vi "Test4_udp.vi"() -> ()   [LabVIEW 2014]
panel:
  out "Numeric":dbl
  in  "stop":bool
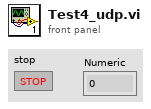
[diagram p1: front panel]
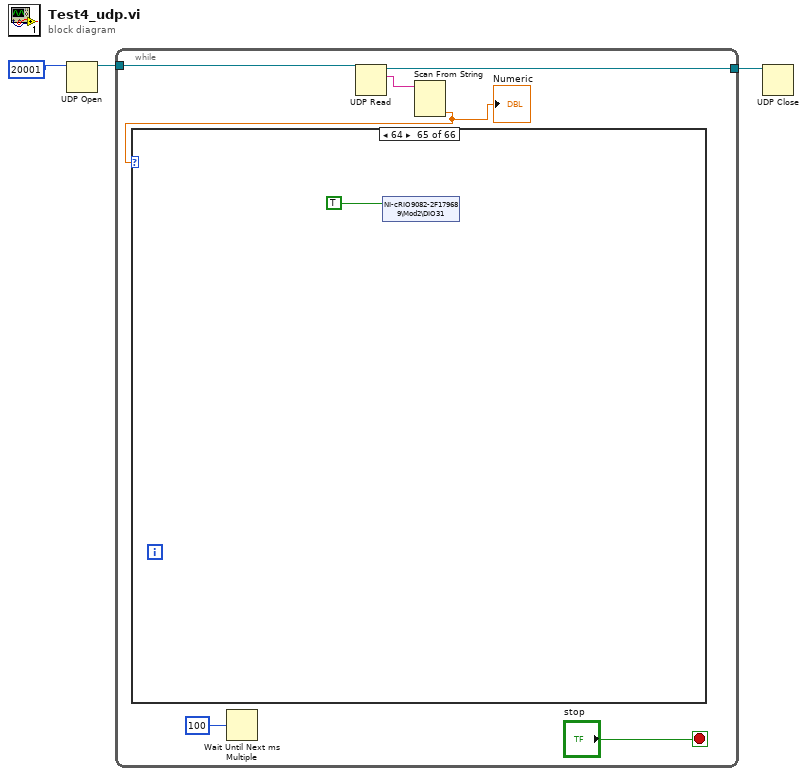
[diagram p0: block diagram]
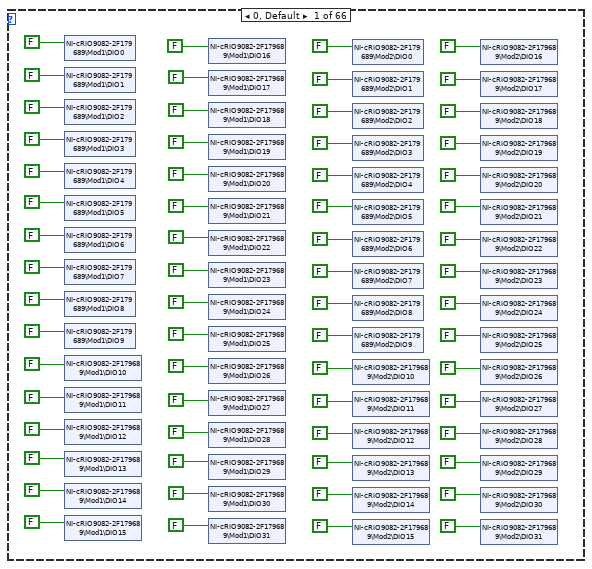
[diagram p2: hidden frame]
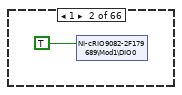
[diagram p3: hidden frame]
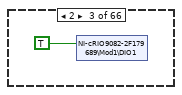
[diagram p4: hidden frame]
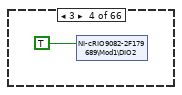
[diagram p5: hidden frame]
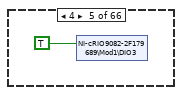
[diagram p6: hidden frame]
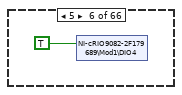
[diagram p7: hidden frame]
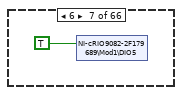
[diagram p8: hidden frame]
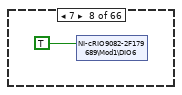
[diagram p9: hidden frame]
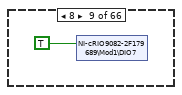
[diagram p10: hidden frame]
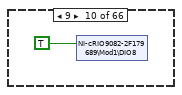
[diagram p11: hidden frame]
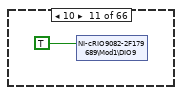
[diagram p12: hidden frame]
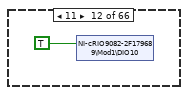
[diagram p13: hidden frame]
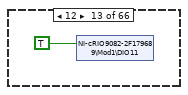
[diagram p14: hidden frame]
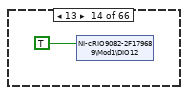
[diagram p15: hidden frame]
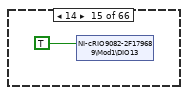
[diagram p16: hidden frame]
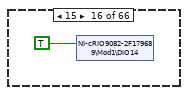
[diagram p17: hidden frame]
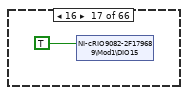
[diagram p18: hidden frame]
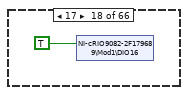
[diagram p19: hidden frame]
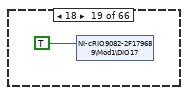
[diagram p20: hidden frame]
diagram:
  n1 = UDP Open(11:u16 20001 ("port")) -> (port=w2:refnum<k16>)  [unwired: 4 in, 2 out]
  n2 = while {
    tunnel: w2 -> [w6]
    tunnel: [w5] -> w1
    stop <- "stop" stop-if-true
    n3 = Wait Until Next ms Multiple(millisecond multiple=u32 100) -> ()  [unwired: 1 out]
    n4 = UDP Read(connection ID=w6) -> (data out=w9:string, 3:w5:refnum<k16>)  [unwired: 3 in, 3 out]
    n5 = Scan From String(input string=w9) -> (output 1=w4:dbl)  [unwired: 4 in, 3 out]
    "Numeric" <- w4
    n6 = case shown="64" w4 {
      frame 0, Default {
        n7 = shared-variable "NI-cRIO9082-2F179689\\Mod1\\DIO0"(FALSE) -> ()  [unwired: 1 in, 1 out]
        n8 = shared-variable "NI-cRIO9082-2F179689\\Mod1\\DIO1"(FALSE) -> ()  [unwired: 1 in, 1 out]
        n9 = shared-variable "NI-cRIO9082-2F179689\\Mod1\\DIO2"(FALSE) -> ()  [unwired: 1 in, 1 out]
        n10 = shared-variable "NI-cRIO9082-2F179689\\Mod1\\DIO3"(FALSE) -> ()  [unwired: 1 in, 1 out]
        n11 = shared-variable "NI-cRIO9082-2F179689\\Mod1\\DIO4"(FALSE) -> ()  [unwired: 1 in, 1 out]
        n12 = shared-variable "NI-cRIO9082-2F179689\\Mod1\\DIO5"(FALSE) -> ()  [unwired: 1 in, 1 out]
        n13 = shared-variable "NI-cRIO9082-2F179689\\Mod1\\DIO6"(FALSE) -> ()  [unwired: 1 in, 1 out]
        n14 = shared-variable "NI-cRIO9082-2F179689\\Mod1\\DIO7"(FALSE) -> ()  [unwired: 1 in, 1 out]
        n15 = shared-variable "NI-cRIO9082-2F179689\\Mod1\\DIO8"(FALSE) -> ()  [unwired: 1 in, 1 out]
        n16 = shared-variable "NI-cRIO9082-2F179689\\Mod1\\DIO9"(FALSE) -> ()  [unwired: 1 in, 1 out]
        n17 = shared-variable "NI-cRIO9082-2F179689\\Mod1\\DIO10"(FALSE) -> ()  [unwired: 1 in, 1 out]
        n18 = shared-variable "NI-cRIO9082-2F179689\\Mod1\\DIO11"(FALSE) -> ()  [unwired: 1 in, 1 out]
        n19 = shared-variable "NI-cRIO9082-2F179689\\Mod1\\DIO12"(FALSE) -> ()  [unwired: 1 in, 1 out]
        n20 = shared-variable "NI-cRIO9082-2F179689\\Mod1\\DIO13"(FALSE) -> ()  [unwired: 1 in, 1 out]
        n21 = shared-variable "NI-cRIO9082-2F179689\\Mod1\\DIO14"(FALSE) -> ()  [unwired: 1 in, 1 out]
        n22 = shared-variable "NI-cRIO9082-2F179689\\Mod1\\DIO15"(FALSE) -> ()  [unwired: 1 in, 1 out]
        n23 = shared-variable "NI-cRIO9082-2F179689\\Mod1\\DIO16"(FALSE) -> ()  [unwired: 1 in, 1 out]
        n24 = shared-variable "NI-cRIO9082-2F179689\\Mod1\\DIO17"(FALSE) -> ()  [unwired: 1 in, 1 out]
        n25 = shared-variable "NI-cRIO9082-2F179689\\Mod1\\DIO18"(FALSE) -> ()  [unwired: 1 in, 1 out]
        n26 = shared-variable "NI-cRIO9082-2F179689\\Mod1\\DIO19"(FALSE) -> ()  [unwired: 1 in, 1 out]
        n27 = shared-variable "NI-cRIO9082-2F179689\\Mod1\\DIO20"(FALSE) -> ()  [unwired: 1 in, 1 out]
        n28 = shared-variable "NI-cRIO9082-2F179689\\Mod1\\DIO21"(FALSE) -> ()  [unwired: 1 in, 1 out]
        n29 = shared-variable "NI-cRIO9082-2F179689\\Mod1\\DIO22"(FALSE) -> ()  [unwired: 1 in, 1 out]
        n30 = shared-variable "NI-cRIO9082-2F179689\\Mod1\\DIO23"(FALSE) -> ()  [unwired: 1 in, 1 out]
        n31 = shared-variable "NI-cRIO9082-2F179689\\Mod1\\DIO24"(FALSE) -> ()  [unwired: 1 in, 1 out]
        n32 = shared-variable "NI-cRIO9082-2F179689\\Mod1\\DIO25"(FALSE) -> ()  [unwired: 1 in, 1 out]
        n33 = shared-variable "NI-cRIO9082-2F179689\\Mod1\\DIO26"(FALSE) -> ()  [unwired: 1 in, 1 out]
        n34 = shared-variable "NI-cRIO9082-2F179689\\Mod1\\DIO27"(FALSE) -> ()  [unwired: 1 in, 1 out]
        n35 = shared-variable "NI-cRIO9082-2F179689\\Mod1\\DIO28"(FALSE) -> ()  [unwired: 1 in, 1 out]
        n36 = shared-variable "NI-cRIO9082-2F179689\\Mod1\\DIO29"(FALSE) -> ()  [unwired: 1 in, 1 out]
        n37 = shared-variable "NI-cRIO9082-2F179689\\Mod1\\DIO30"(FALSE) -> ()  [unwired: 1 in, 1 out]
        n38 = shared-variable "NI-cRIO9082-2F179689\\Mod1\\DIO31"(FALSE) -> ()  [unwired: 1 in, 1 out]
        n39 = shared-variable "NI-cRIO9082-2F179689\\Mod2\\DIO0"(FALSE) -> ()  [unwired: 1 in, 1 out]
        n40 = shared-variable "NI-cRIO9082-2F179689\\Mod2\\DIO1"(FALSE) -> ()  [unwired: 1 in, 1 out]
        n41 = shared-variable "NI-cRIO9082-2F179689\\Mod2\\DIO2"(FALSE) -> ()  [unwired: 1 in, 1 out]
        n42 = shared-variable "NI-cRIO9082-2F179689\\Mod2\\DIO3"(FALSE) -> ()  [unwired: 1 in, 1 out]
        n43 = shared-variable "NI-cRIO9082-2F179689\\Mod2\\DIO4"(FALSE) -> ()  [unwired: 1 in, 1 out]
        n44 = shared-variable "NI-cRIO9082-2F179689\\Mod2\\DIO5"(FALSE) -> ()  [unwired: 1 in, 1 out]
        n45 = shared-variable "NI-cRIO9082-2F179689\\Mod2\\DIO6"(FALSE) -> ()  [unwired: 1 in, 1 out]
        n46 = shared-variable "NI-cRIO9082-2F179689\\Mod2\\DIO7"(FALSE) -> ()  [unwired: 1 in, 1 out]
        n47 = shared-variable "NI-cRIO9082-2F179689\\Mod2\\DIO8"(FALSE) -> ()  [unwired: 1 in, 1 out]
        n48 = shared-variable "NI-cRIO9082-2F179689\\Mod2\\DIO9"(FALSE) -> ()  [unwired: 1 in, 1 out]
        n49 = shared-variable "NI-cRIO9082-2F179689\\Mod2\\DIO10"(FALSE) -> ()  [unwired: 1 in, 1 out]
        n50 = shared-variable "NI-cRIO9082-2F179689\\Mod2\\DIO11"(FALSE) -> ()  [unwired: 1 in, 1 out]
        n51 = shared-variable "NI-cRIO9082-2F179689\\Mod2\\DIO12"(FALSE) -> ()  [unwired: 1 in, 1 out]
        n52 = shared-variable "NI-cRIO9082-2F179689\\Mod2\\DIO13"(FALSE) -> ()  [unwired: 1 in, 1 out]
        n53 = shared-variable "NI-cRIO9082-2F179689\\Mod2\\DIO14"(FALSE) -> ()  [unwired: 1 in, 1 out]
        n54 = shared-variable "NI-cRIO9082-2F179689\\Mod2\\DIO15"(FALSE) -> ()  [unwired: 1 in, 1 out]
        n55 = shared-variable "NI-cRIO9082-2F179689\\Mod2\\DIO16"(FALSE) -> ()  [unwired: 1 in, 1 out]
        n56 = shared-variable "NI-cRIO9082-2F179689\\Mod2\\DIO17"(FALSE) -> ()  [unwired: 1 in, 1 out]
        n57 = shared-variable "NI-cRIO9082-2F179689\\Mod2\\DIO18"(FALSE) -> ()  [unwired: 1 in, 1 out]
        n58 = shared-variable "NI-cRIO9082-2F179689\\Mod2\\DIO19"(FALSE) -> ()  [unwired: 1 in, 1 out]
        n59 = shared-variable "NI-cRIO9082-2F179689\\Mod2\\DIO20"(FALSE) -> ()  [unwired: 1 in, 1 out]
        n60 = shared-variable "NI-cRIO9082-2F179689\\Mod2\\DIO21"(FALSE) -> ()  [unwired: 1 in, 1 out]
        n61 = shared-variable "NI-cRIO9082-2F179689\\Mod2\\DIO22"(FALSE) -> ()  [unwired: 1 in, 1 out]
        n62 = shared-variable "NI-cRIO9082-2F179689\\Mod2\\DIO23"(FALSE) -> ()  [unwired: 1 in, 1 out]
        n63 = shared-variable "NI-cRIO9082-2F179689\\Mod2\\DIO24"(FALSE) -> ()  [unwired: 1 in, 1 out]
        n64 = shared-variable "NI-cRIO9082-2F179689\\Mod2\\DIO25"(FALSE) -> ()  [unwired: 1 in, 1 out]
        n65 = shared-variable "NI-cRIO9082-2F179689\\Mod2\\DIO26"(FALSE) -> ()  [unwired: 1 in, 1 out]
        n66 = shared-variable "NI-cRIO9082-2F179689\\Mod2\\DIO27"(FALSE) -> ()  [unwired: 1 in, 1 out]
        n67 = shared-variable "NI-cRIO9082-2F179689\\Mod2\\DIO28"(FALSE) -> ()  [unwired: 1 in, 1 out]
        n68 = shared-variable "NI-cRIO9082-2F179689\\Mod2\\DIO29"(FALSE) -> ()  [unwired: 1 in, 1 out]
        n69 = shared-variable "NI-cRIO9082-2F179689\\Mod2\\DIO30"(FALSE) -> ()  [unwired: 1 in, 1 out]
        n70 = shared-variable "NI-cRIO9082-2F179689\\Mod2\\DIO31"(FALSE) -> ()  [unwired: 1 in, 1 out]
      }
      frame 1 {
        n71 = shared-variable "NI-cRIO9082-2F179689\\Mod1\\DIO0"(TRUE) -> ()  [unwired: 1 in, 1 out]
      }
      frame 2 {
        n72 = shared-variable "NI-cRIO9082-2F179689\\Mod1\\DIO1"(TRUE) -> ()  [unwired: 1 in, 1 out]
      }
      frame 3 {
        n73 = shared-variable "NI-cRIO9082-2F179689\\Mod1\\DIO2"(TRUE) -> ()  [unwired: 1 in, 1 out]
      }
      frame 4 {
        n74 = shared-variable "NI-cRIO9082-2F179689\\Mod1\\DIO3"(TRUE) -> ()  [unwired: 1 in, 1 out]
      }
      frame 5 {
        n75 = shared-variable "NI-cRIO9082-2F179689\\Mod1\\DIO4"(TRUE) -> ()  [unwired: 1 in, 1 out]
      }
      frame 6 {
        n76 = shared-variable "NI-cRIO9082-2F179689\\Mod1\\DIO5"(TRUE) -> ()  [unwired: 1 in, 1 out]
      }
      frame 7 {
        n77 = shared-variable "NI-cRIO9082-2F179689\\Mod1\\DIO6"(TRUE) -> ()  [unwired: 1 in, 1 out]
      }
      frame 8 {
        n78 = shared-variable "NI-cRIO9082-2F179689\\Mod1\\DIO7"(TRUE) -> ()  [unwired: 1 in, 1 out]
      }
      frame 9 {
        n79 = shared-variable "NI-cRIO9082-2F179689\\Mod1\\DIO8"(TRUE) -> ()  [unwired: 1 in, 1 out]
      }
      frame 10 {
        n80 = shared-variable "NI-cRIO9082-2F179689\\Mod1\\DIO9"(TRUE) -> ()  [unwired: 1 in, 1 out]
      }
      frame 11 {
        n81 = shared-variable "NI-cRIO9082-2F179689\\Mod1\\DIO10"(TRUE) -> ()  [unwired: 1 in, 1 out]
      }
      frame 12 {
        n82 = shared-variable "NI-cRIO9082-2F179689\\Mod1\\DIO11"(TRUE) -> ()  [unwired: 1 in, 1 out]
      }
      frame 13 {
        n83 = shared-variable "NI-cRIO9082-2F179689\\Mod1\\DIO12"(TRUE) -> ()  [unwired: 1 in, 1 out]
      }
      frame 14 {
        n84 = shared-variable "NI-cRIO9082-2F179689\\Mod1\\DIO13"(TRUE) -> ()  [unwired: 1 in, 1 out]
      }
      frame 15 {
        n85 = shared-variable "NI-cRIO9082-2F179689\\Mod1\\DIO14"(TRUE) -> ()  [unwired: 1 in, 1 out]
      }
      frame 16 {
        n86 = shared-variable "NI-cRIO9082-2F179689\\Mod1\\DIO15"(TRUE) -> ()  [unwired: 1 in, 1 out]
      }
      frame 17 {
        n87 = shared-variable "NI-cRIO9082-2F179689\\Mod1\\DIO16"(TRUE) -> ()  [unwired: 1 in, 1 out]
      }
      frame 18 {
        n88 = shared-variable "NI-cRIO9082-2F179689\\Mod1\\DIO17"(TRUE) -> ()  [unwired: 1 in, 1 out]
      }
      frame 19 {
        n89 = shared-variable "NI-cRIO9082-2F179689\\Mod1\\DIO18"(TRUE) -> ()  [unwired: 1 in, 1 out]
      }
      frame 20 {
        n90 = shared-variable "NI-cRIO9082-2F179689\\Mod1\\DIO19"(TRUE) -> ()  [unwired: 1 in, 1 out]
      }
      frame 21 {
        n91 = shared-variable "NI-cRIO9082-2F179689\\Mod1\\DIO20"(TRUE) -> ()  [unwired: 1 in, 1 out]
      }
      frame 22 {
        n92 = shared-variable "NI-cRIO9082-2F179689\\Mod1\\DIO21"(TRUE) -> ()  [unwired: 1 in, 1 out]
      }
      frame 23 {
        n93 = shared-variable "NI-cRIO9082-2F179689\\Mod1\\DIO22"(TRUE) -> ()  [unwired: 1 in, 1 out]
      }
      frame 24 {
        n94 = shared-variable "NI-cRIO9082-2F179689\\Mod1\\DIO23"(TRUE) -> ()  [unwired: 1 in, 1 out]
      }
      frame 25 {
        n95 = shared-variable "NI-cRIO9082-2F179689\\Mod1\\DIO24"(TRUE) -> ()  [unwired: 1 in, 1 out]
      }
      frame 26 {
        n96 = shared-variable "NI-cRIO9082-2F179689\\Mod1\\DIO25"(TRUE) -> ()  [unwired: 1 in, 1 out]
      }
      frame 27 {
        n97 = shared-variable "NI-cRIO9082-2F179689\\Mod1\\DIO26"(TRUE) -> ()  [unwired: 1 in, 1 out]
      }
      frame 28 {
        n98 = shared-variable "NI-cRIO9082-2F179689\\Mod1\\DIO27"(TRUE) -> ()  [unwired: 1 in, 1 out]
      }
      frame 29 {
        n99 = shared-variable "NI-cRIO9082-2F179689\\Mod1\\DIO28"(TRUE) -> ()  [unwired: 1 in, 1 out]
      }
      frame 30 {
        n100 = shared-variable "NI-cRIO9082-2F179689\\Mod1\\DIO29"(TRUE) -> ()  [unwired: 1 in, 1 out]
      }
      frame 31 {
        n101 = shared-variable "NI-cRIO9082-2F179689\\Mod1\\DIO30"(TRUE) -> ()  [unwired: 1 in, 1 out]
      }
      frame 32 {
        n102 = shared-variable "NI-cRIO9082-2F179689\\Mod1\\DIO31"(TRUE) -> ()  [unwired: 1 in, 1 out]
      }
      frame 33 {
        n103 = shared-variable "NI-cRIO9082-2F179689\\Mod2\\DIO0"(TRUE) -> ()  [unwired: 1 in, 1 out]
      }
      frame 34 {
        n104 = shared-variable "NI-cRIO9082-2F179689\\Mod2\\DIO1"(TRUE) -> ()  [unwired: 1 in, 1 out]
      }
      frame 35 {
        n105 = shared-variable "NI-cRIO9082-2F179689\\Mod2\\DIO2"(TRUE) -> ()  [unwired: 1 in, 1 out]
      }
      frame 36 {
        n106 = shared-variable "NI-cRIO9082-2F179689\\Mod2\\DIO3"(TRUE) -> ()  [unwired: 1 in, 1 out]
      }
      frame 37 {
        n107 = shared-variable "NI-cRIO9082-2F179689\\Mod2\\DIO4"(TRUE) -> ()  [unwired: 1 in, 1 out]
      }
      frame 38 {
        n108 = shared-variable "NI-cRIO9082-2F179689\\Mod2\\DIO5"(TRUE) -> ()  [unwired: 1 in, 1 out]
      }
      frame 39 {
        n109 = shared-variable "NI-cRIO9082-2F179689\\Mod2\\DIO6"(TRUE) -> ()  [unwired: 1 in, 1 out]
      }
      frame 40 {
        n110 = shared-variable "NI-cRIO9082-2F179689\\Mod2\\DIO7"(TRUE) -> ()  [unwired: 1 in, 1 out]
      }
      frame 41 {
        n111 = shared-variable "NI-cRIO9082-2F179689\\Mod2\\DIO8"(TRUE) -> ()  [unwired: 1 in, 1 out]
      }
      frame 42 {
        n112 = shared-variable "NI-cRIO9082-2F179689\\Mod2\\DIO9"(TRUE) -> ()  [unwired: 1 in, 1 out]
      }
      frame 43 {
        n113 = shared-variable "NI-cRIO9082-2F179689\\Mod2\\DIO10"(TRUE) -> ()  [unwired: 1 in, 1 out]
      }
      frame 44 {
        n114 = shared-variable "NI-cRIO9082-2F179689\\Mod2\\DIO11"(TRUE) -> ()  [unwired: 1 in, 1 out]
      }
      frame 45 {
        n115 = shared-variable "NI-cRIO9082-2F179689\\Mod2\\DIO12"(TRUE) -> ()  [unwired: 1 in, 1 out]
      }
      frame 46 {
        n116 = shared-variable "NI-cRIO9082-2F179689\\Mod2\\DIO13"(TRUE) -> ()  [unwired: 1 in, 1 out]
      }
      frame 47 {
        n117 = shared-variable "NI-cRIO9082-2F179689\\Mod2\\DIO14"(TRUE) -> ()  [unwired: 1 in, 1 out]
      }
      frame 48 {
        n118 = shared-variable "NI-cRIO9082-2F179689\\Mod2\\DIO15"(TRUE) -> ()  [unwired: 1 in, 1 out]
      }
      frame 49 {
        n119 = shared-variable "NI-cRIO9082-2F179689\\Mod2\\DIO16"(TRUE) -> ()  [unwired: 1 in, 1 out]
      }
      frame 50 {
        n120 = shared-variable "NI-cRIO9082-2F179689\\Mod2\\DIO17"(TRUE) -> ()  [unwired: 1 in, 1 out]
      }
      frame 51 {
        n121 = shared-variable "NI-cRIO9082-2F179689\\Mod2\\DIO18"(TRUE) -> ()  [unwired: 1 in, 1 out]
      }
      frame 52 {
        n122 = shared-variable "NI-cRIO9082-2F179689\\Mod2\\DIO19"(TRUE) -> ()  [unwired: 1 in, 1 out]
      }
      frame 53 {
        n123 = shared-variable "NI-cRIO9082-2F179689\\Mod2\\DIO20"(TRUE) -> ()  [unwired: 1 in, 1 out]
      }
      frame 54 {
        n124 = shared-variable "NI-cRIO9082-2F179689\\Mod2\\DIO21"(TRUE) -> ()  [unwired: 1 in, 1 out]
      }
      frame 55 {
        n125 = shared-variable "NI-cRIO9082-2F179689\\Mod2\\DIO22"(TRUE) -> ()  [unwired: 1 in, 1 out]
      }
      frame 56 {
        n126 = shared-variable "NI-cRIO9082-2F179689\\Mod2\\DIO23"(TRUE) -> ()  [unwired: 1 in, 1 out]
      }
      frame 57 {
        n127 = shared-variable "NI-cRIO9082-2F179689\\Mod2\\DIO24"(TRUE) -> ()  [unwired: 1 in, 1 out]
      }
      frame 58 {
        n128 = shared-variable "NI-cRIO9082-2F179689\\Mod2\\DIO25"(TRUE) -> ()  [unwired: 1 in, 1 out]
      }
      frame 59 {
        n129 = shared-variable "NI-cRIO9082-2F179689\\Mod2\\DIO26"(TRUE) -> ()  [unwired: 1 in, 1 out]
      }
      frame 60 {
        n130 = shared-variable "NI-cRIO9082-2F179689\\Mod2\\DIO27"(TRUE) -> ()  [unwired: 1 in, 1 out]
      }
      frame 61 {
        n131 = shared-variable "NI-cRIO9082-2F179689\\Mod2\\DIO28"(TRUE) -> ()  [unwired: 1 in, 1 out]
      }
      frame 62 {
        n132 = shared-variable "NI-cRIO9082-2F179689\\Mod2\\DIO29"(TRUE) -> ()  [unwired: 1 in, 1 out]
      }
      frame 63 {
        n133 = shared-variable "NI-cRIO9082-2F179689\\Mod2\\DIO30"(TRUE) -> ()  [unwired: 1 in, 1 out]
      }
      frame 64 {
        n134 = shared-variable "NI-cRIO9082-2F179689\\Mod2\\DIO31"(TRUE) -> ()  [unwired: 1 in, 1 out]
      }
      frame 65 {
        n135 = shared-variable "NI-cRIO9082-2F179689\\Mod2\\DIO0"(TRUE) -> ()  [unwired: 1 in, 1 out]
      }
    }
  }
  n136 = UDP Close(connection ID=w1) -> ()  [unwired: 1 in, 2 out]
